vi "Unit Test - Copy Specified State.vi"() -> (3 "Array":T1(array[cluster])=[{"state"="Idle", "error out"={"status"=FALSE, "code"=0, "source"=""}, "Execution:State"=enum."Idle"}, {"state"="CSM Documentation", "error out"={"status"=FALSE, "code"=0, "source"=""}, "Execution:State"=enum."Idle"}, {"state"="VI Reference", "error out"={"status"=FALSE, "code"=0, "source"=""}, "Execution:State"=enum."Idle"}, {"state"="Error Handler", "error out"={"status"=FALSE, "code"=0, "source"=""}, "Execution:State"=enum."Bad"}, {"state"="Critical Error", "error out"={"status"=FALSE, "code"=0, "source"=""}, "Execution:State"=enum."Idle"}, {"state"="Target Timeout Error", "error out"={"status"=FALSE, "code"=0, "source"=""}, "Execution:State"=enum."Idle"}, {"state"="Target Error", "error out"={"status"=FALSE, "code"=0, "source"=""}, "Execution:State"=enum."Idle"}, {"state"="Async Response", "error out"={"status"=FALSE, "code"=0, "source"=""}, "Execution:State"=enum."Idle"}, {"state"="Response", "error out"={"status"=FALSE, "code"=0, "source"=""}, "Execution:State"=enum."Idle"}, {"state"="Async Message Posted", "error out"={"status"=FALSE, "code"=0, "source"=""}, "Execution:State"=enum."Idle"}, {"state"="Initialize Core Data", "error out"={"status"=FALSE, "code"=0, "source"=""}, "Execution:State"=enum."Idle"}, {"state"="Exit", "error out"={"status"=FALSE, "code"=0, "source"=""}, "Execution:State"=enum."Idle"}, {"state"="Data: Initialize", "error out"={"status"=FALSE, "code"=0, "source"=""}, "Execution:State"=enum."Idle"}, {"state"="Data: Update Indicators", "error out"={"status"=FALSE, "code"=0, "source"=""}, "Execution:State"=enum."Idle"}, {"state"="Data: Cleanup", "error out"={"status"=FALSE, "code"=0, "source"=""}, "Execution:State"=enum."Idle"}, {"state"="Macro: Initialize", "error out"={"status"=FALSE, "code"=0, "source"=""}, "Execution:State"=enum."Idle"}, {"state"="Macro: Exit", "error out"={"status"=FALSE, "code"=0, "source"=""}, "Execution:State"=enum."Idle"}, {"state"="API: API1", "error out"={"status"=FALSE, "code"=0, "source"=""}, "Execution:State"=enum."Idle"}, {"state"="API: API2", "error out"={"status"=FALSE, "code"=0, "source"=""}, "Execution:State"=enum."Idle"}, {"state"="Action: action1", "error out"={"status"=FALSE, "code"=0, "source"=""}, "Execution:State"=enum."Idle"}, {"state"="Action: action2", "error out"={"status"=FALSE, "code"=0, "source"=""}, "Execution:State"=enum."Idle"}])   [LabVIEW 2017, in "testcase-csmhelper.lvclass"]
uses:
  testcase-csmhelper.lvclass
  src/user.lib/_NEVSTOP/Communicable State Machine(CSM)/_csmHelper/CSM-Helper.lvclass/CSM-Helper.ctl
  src/user.lib/_NEVSTOP/Communicable State Machine(CSM)/_csmHelper/Properties/Read VI Ref.vi
  src/user.lib/_NEVSTOP/Communicable State Machine(CSM)/_csmHelper/API/Create From VI Reference.vi
  src/user.lib/_NEVSTOP/Communicable State Machine(CSM)/_csmHelper/API/Open Block Diagram.vi
  src/user.lib/_NEVSTOP/Communicable State Machine(CSM)/_csmHelper/API/Start Undo.vi
  src/user.lib/_NEVSTOP/Communicable State Machine(CSM)/_csmHelper/API/Copy State.vi
  src/user.lib/_NEVSTOP/Communicable State Machine(CSM)/_csmHelper/API/Stop Undo.vi
  src/user.lib/_NEVSTOP/Communicable State Machine(CSM)/_csmHelper/API/Undo.vi
  src/user.lib/_NEVSTOP/Communicable State Machine(CSM)/_csmHelper/API/Destroy.vi
  src/user.lib/_NEVSTOP/Communicable State Machine(CSM)/_csmHelper/CSM-Helper.lvclass
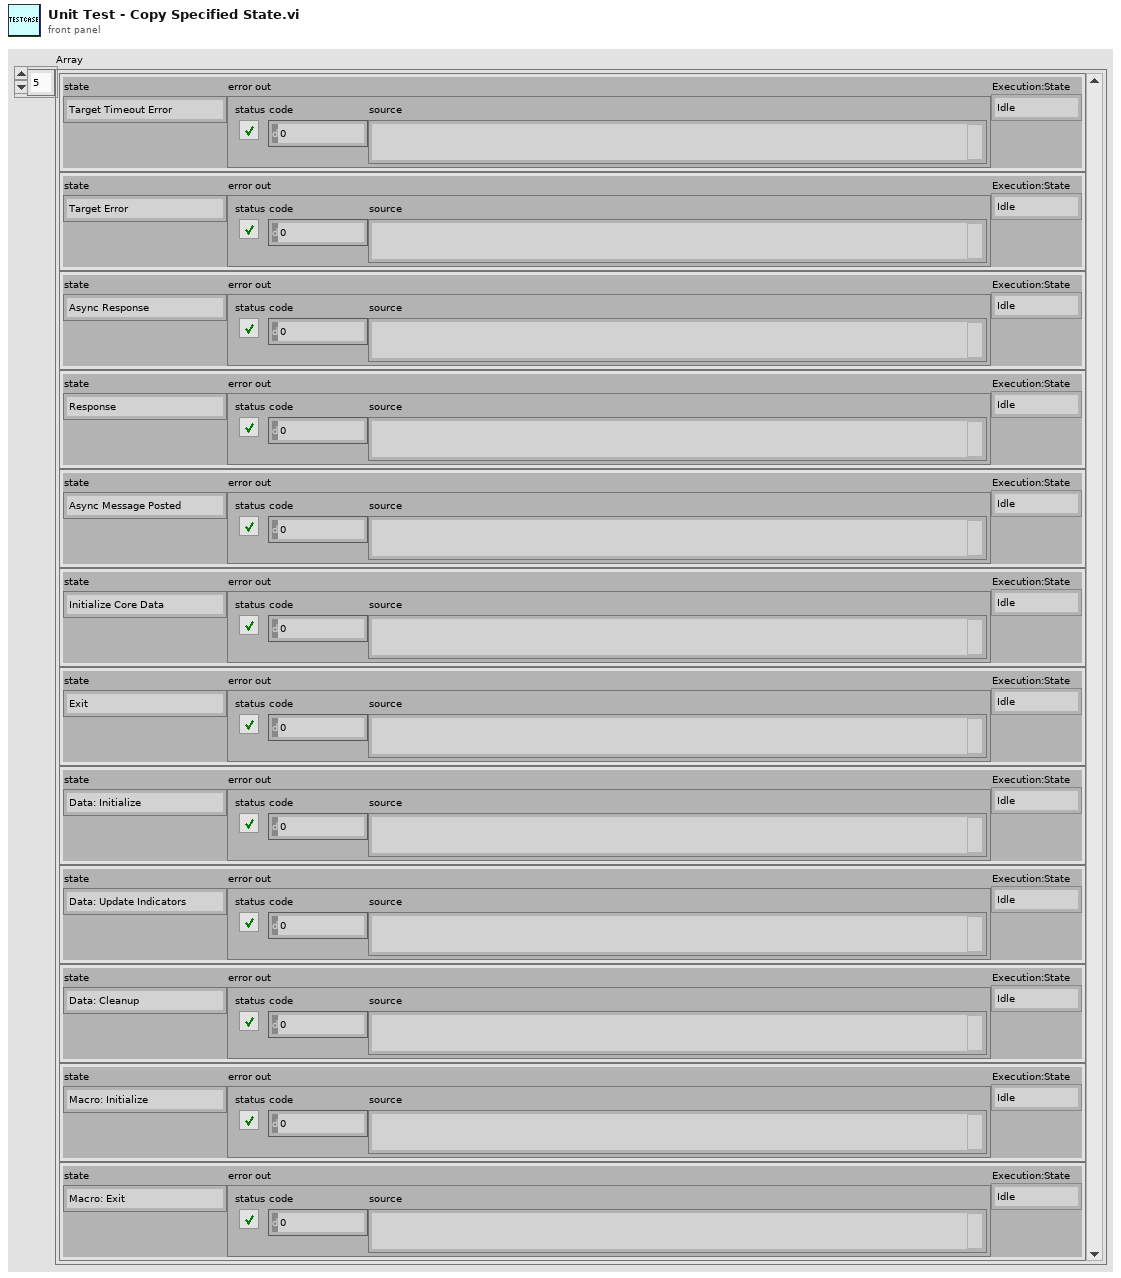
[diagram p1: front panel]
types:
  T1 = cluster{"state":string, "error out":errorcluster, "Execution:State":enum32{"Bad", "Idle", "Run top level", "Running"}}[]
  T2 = enum32{"Bad", "Idle", "Run top level", "Running"}
  T3 = cluster{string, "error out":errorcluster, "Exec.State":enum32{"Bad", "Idle", "Run top level", "Running"}}
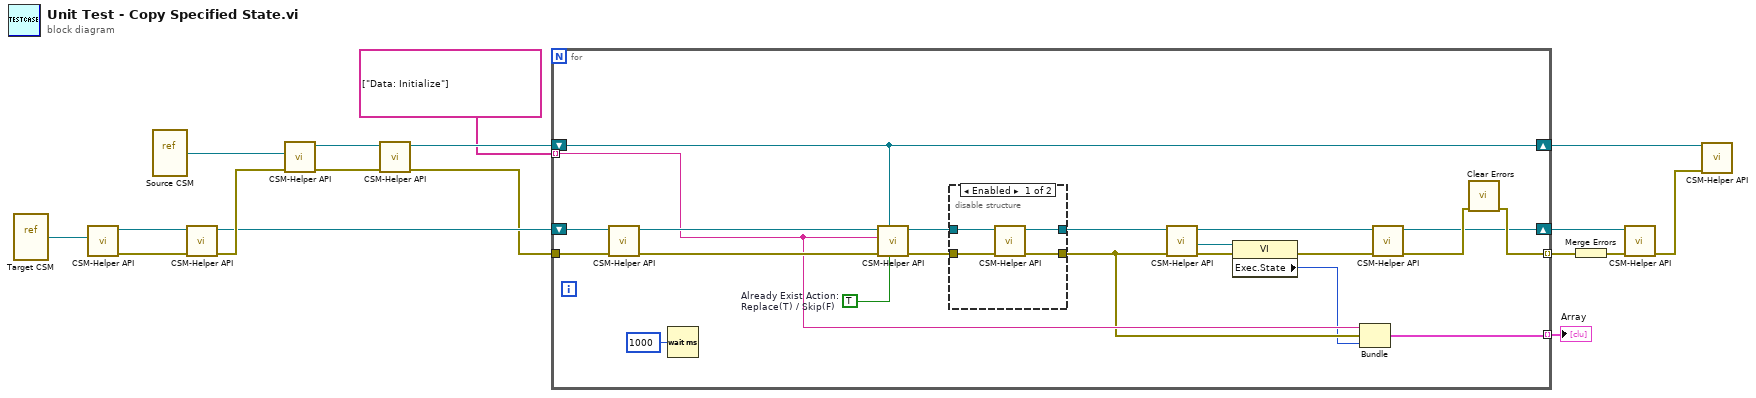
[diagram p0: block diagram]
diagram:
  n1 = vi-ref "Target CSM.vi"() -> (w16:refnum<vi>)
  n2 = call-poly "CSM-Helper API.vi"("VI"=w16) -> ("error out"=w13:errorcluster, "CSM-Helper.lvclass"=w12:refnum<class "CSM-Helper.lvclass">)  [unwired: 9 in]
  n3 = vi-ref "Source CSM.vi"() -> (w17:refnum<vi>)
  n4 = call-poly "CSM-Helper API.vi"("error in (no error)"=w13, "CSM-Helper in"=w12) -> ("error out"=w9:errorcluster, "CSM-Helper out"=w8:refnum<class "CSM-Helper.lvclass">)  [unwired: 8 in]
  n5 = call-poly "CSM-Helper API.vi"("error in (no error)"=w9, "VI"=w17) -> ("error out"=w10:errorcluster, "CSM-Helper.lvclass"=w11:refnum<class "CSM-Helper.lvclass">)  [unwired: 8 in]
  n6 = call-poly "CSM-Helper API.vi"("error in (no error)"=w10, "CSM-Helper in"=w11) -> ("error out"=w2:errorcluster, "CSM-Helper out"=w3:refnum<class "CSM-Helper.lvclass">)  [unwired: 8 in]
  n7 = for {
    shift-right: [w26] -> w15
    shift-left: w8 -> [w37]
    shift-right: [w32] -> w6
    shift-left: w3 -> [w32]
    tunnel: string[] ["Data: Initialize"] ("Value") -> [w30] mode=indexing
    tunnel: w2 -> [w36]
    tunnel: [w31] -> w14 mode=indexing
    tunnel: [w29] -> w4 mode=indexing
    w18 = TRUE  # Already Exist Action: Replace(T) / Skip(F)
    n8 = call-poly "CSM-Helper API.vi"("error in (no error)"=w36, "CSM-Helper in"=w37) -> ("error out"=w35:errorcluster, "CSM-Helper out"=w34:refnum<class "CSM-Helper.lvclass">)  [unwired: 8 in]
    n9 = Wait (ms)(milliseconds to wait=u32 1000) -> ()  [unwired: 1 out]
    n10 = call-poly "CSM-Helper API.vi"("Already Exist Action:\nReplace(T) / Skip(F)"=w18, "SourceCSM"=w32, "error in (no error)"=w35, "Case"=w30, "CSM-Helper.lvclass"=w34) -> ("error out"=w33:errorcluster, "CSM-Helper out 2"=w38:refnum<class "CSM-Helper.lvclass">)  [unwired: 5 in]
    n11 = disable-structure shown="Enabled" {
      disable-tunnel: [w42 w44] -> w24
      disable-tunnel: w33 -> [w41 w43]
      disable-tunnel: [w40 w43] -> w25
      disable-tunnel: w38 -> [w39 w44]
      frame Enabled {
        n12 = call-poly "CSM-Helper API.vi"("error in (no error)"=w41, "CSM-Helper in"=w39) -> ("error out"=w40:errorcluster, "CSM-Helper out"=w42:refnum<class "CSM-Helper.lvclass">)  [unwired: 8 in]
      }
      frame Disabled {
      }
    }
    n13 = call-poly "CSM-Helper API.vi"("error in (no error)"=w25, "CSM-Helper in"=w24) -> ("error out"=w22:errorcluster, "VI"=w20:refnum<vi>, "CSM-Helper out"=w23:refnum<class "CSM-Helper.lvclass">)  [unwired: 7 in]
    n14 = property class="VI"(reference=w20, error in=w22) -> (error out=w21:errorcluster, "Exec.State"=w19:T2)  [unwired: 1 out]
    n15 = Bundle(w30, "error out"=w25, "Exec.State"=w19) -> (w29:T3)  [unwired: 1 in]
    n16 = call-poly "CSM-Helper API.vi"("error in (no error)"=w21, "CSM-Helper in"=w23) -> ("error out"=w27:errorcluster, "CSM-Helper out"=w26:refnum<class "CSM-Helper.lvclass">)  [unwired: 8 in]
    n17 = call <vilib>:"Clear Errors.vi"("error in (no error)"=w27) -> ("error out"=w31:errorcluster)  [unwired: 5 in, 1 out]
  }
  "Array" <- w4
  n18 = Merge Errors(w14) -> (w5:errorcluster)
  n19 = call-poly "CSM-Helper API.vi"("error in (no error)"=w5, "CSM-Helper in"=w15) -> ("error out"=w7:errorcluster)  [unwired: 8 in, 1 out]
  n20 = call-poly "CSM-Helper API.vi"("error in (no error)"=w7, "CSM-Helper in"=w6) -> ()  [unwired: 8 in, 2 out]
